vi "unused_shift.vi"(8 "error in (no error)":errorcluster, 9 "deltaY[pixel]":i32, 10 "deltaX_[pixel]":i32, 11 "GObject in":refnum<class "Generic.lvclass">) -> (0 "error out":errorcluster, 3 "GObject out":refnum<class "Generic.lvclass">)   [LabVIEW 2023]
uses:
  Generic.lvclass
  Generic.lvclass/Generic.ctl
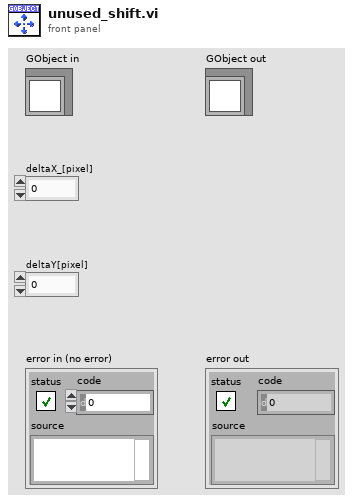
[diagram p1: front panel]
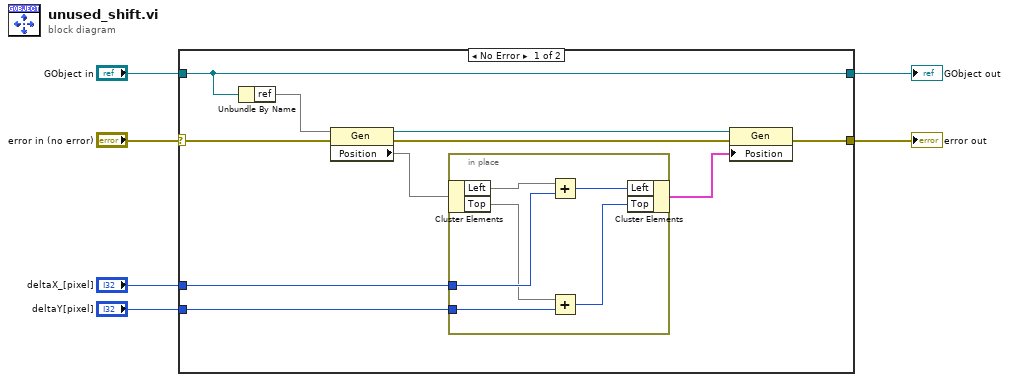
[diagram p0: block diagram]
diagram:
  n1 = case shown="No Error" "error in (no error)" {
    selector: "error in (no error)" -> [w12 w24]
    tunnel: [w11 w24] -> w5
    tunnel: [w16 w23] -> w3
    tunnel: "GObject in" -> [w16 w23]
    tunnel: "deltaX_[pixel]" -> [w8 _]
    tunnel: "deltaY[pixel]" -> [w7 _]
    frame No Error {
      n2 = Unbundle By Name(w16) -> ("ref"=w15)
      n3 = property class="Gen"(reference=w15, error in=w12) -> (reference out=w14:refnum<vi>, error out=w13:errorcluster, "Position"=w10)
      n4 = in-place {
        in-place-border: w8 -> [w21]
        in-place-border: w7 -> [w17]
        n5 = in-place-cluster #1(w10) -> ("Left"=w22, "Top"=w19)
        n6 = Add(x=w22, y=w21) -> (x+y=w20:i32)
        n7 = Add(x=w19, y=w17) -> (x+y=w18:i32)
        n8 = in-place-cluster #1("Left"=w20, "Top"=w18) -> (w9:cluster{})
      }
      n9 = property class="Gen"(reference=w14, error in=w13, "Position"=w9) -> (error out=w11:errorcluster)  [unwired: 1 out]
    }
    frame Error {
    }
  }
  "error out" <- w5
  "GObject out" <- w3
